vi "Convert Dual Tone Prop from String.vi"(8 "error in (no error)":errorcluster, 11 "dual tone properties":string) -> (0 "error out":errorcluster, 3 "dual tone properties":T1)   [LabVIEW 2021, in "AudioGenTypeDefs.lvlib"]
uses:
  AudioGenTypeDefs.lvlib
  dual tone properties.ctl
  dual tone types.ctl
  dual tone properties_JSON.ctl
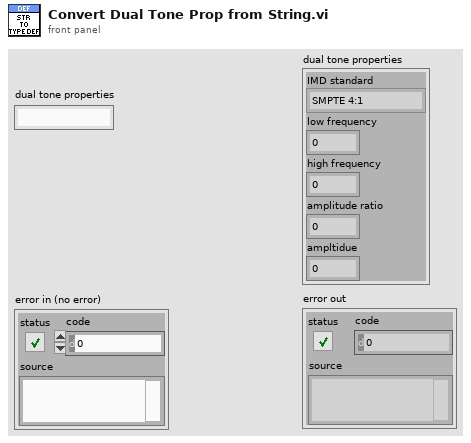
[diagram p1: front panel]
types:
  T1 = typedef "AudioGenTypeDefs.lvlib/dual tone properties.ctl" = cluster{"IMD standard":T2, "low frequency":dbl, "high frequency":dbl, "amplitude ratio":dbl, "ampltidue":dbl}
  T2 = typedef "AudioGenTypeDefs.lvlib/dual tone types.ctl" = enum32{"SMPTE 4:1", "DIN", "CCIF 11k-12k", "CCIF 19k-20k", "Custom"}
  T3 = typedef "AudioGenTypeDefs.lvlib/dual tone properties_JSON.ctl" = cluster{"IMD standard":string, "low frequency":dbl, "high frequency":dbl, "amplitude ratio":dbl, "ampltidue":dbl}
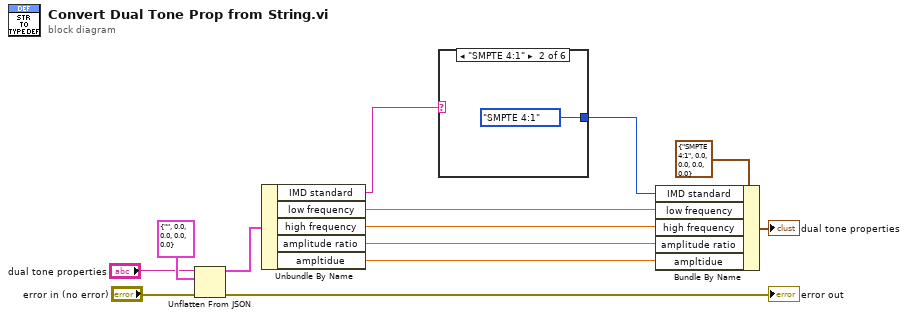
[diagram p0: block diagram]
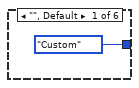
[diagram p2: hidden frame]
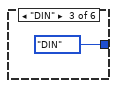
[diagram p3: hidden frame]
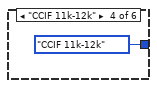
[diagram p4: hidden frame]
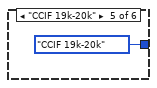
[diagram p5: hidden frame]
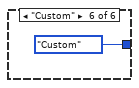
[diagram p6: hidden frame]
diagram:
  n1 = Unflatten From JSON(JSON string="dual tone properties", type and defaults=T3 {"IMD standard"="", "low frequency"=0.0, "high frequency"=0.0, "amplitude ratio"=0.0, "ampltidue"=0.0} ("dual tone properties"), error in (no error)="error in (no error)") -> (value=w8:T3, error out=→"error out":errorcluster)  [unwired: 4 in]
  n2 = Unbundle By Name(w8) -> ("IMD standard"=w2:string, "low frequency"=w7:dbl, "high frequency"=w6:dbl, "amplitude ratio"=w5:dbl, "ampltidue"=w4:dbl)
  n3 = case shown="\"SMPTE 4:1\"" w2 {
    tunnel: [dual_tone_types."Custom" ("IMD standard") dual_tone_types."SMPTE 4:1" ("IMD standard") dual_tone_types."DIN" ("IMD standard") dual_tone_types."CCIF 11k-12k" ("IMD standard") dual_tone_types."CCIF 19k-20k" ("IMD standard") dual_tone_types."Custom" ("IMD standard")] -> w1
    frame "", Default {
    }
    frame "SMPTE 4:1" {
    }
    frame "DIN" {
    }
    frame "CCIF 11k-12k" {
    }
    frame "CCIF 19k-20k" {
    }
    frame "Custom" {
    }
  }
  n4 = Bundle By Name(cluster=T1 {"IMD standard"=enum."SMPTE 4:1", "low frequency"=0.0, "high frequency"=0.0, "amplitude ratio"=0.0, "ampltidue"=0.0} ("dual tone properties"), "IMD standard"=w1, "low frequency"=w7, "high frequency"=w6, "amplitude ratio"=w5, "ampltidue"=w4) -> (→"dual tone properties":T1)
